vi "Untitled 2.vi"() -> ()   [LabVIEW 2018]
panel:
  in  "Action":enum16{"Create", "Fire", "Get", "Destroy"}(ring)=enum."Destroy"
  in  "Error In":errorcluster
  out "error out":errorcluster
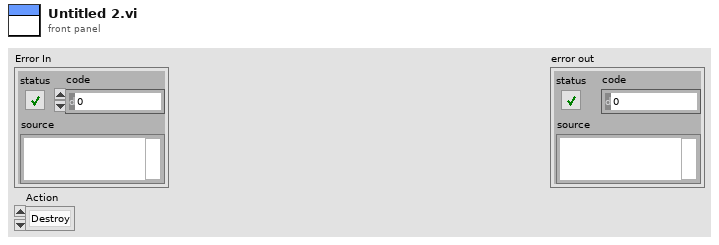
[diagram p1: front panel]
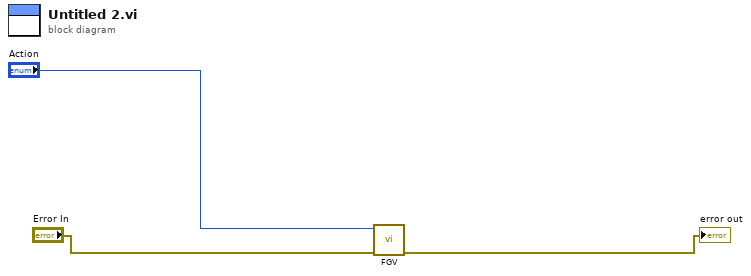
[diagram p0: block diagram]
diagram:
  n1 = call "FGV.vi"("error in"="Error In", 11:"Action") -> ("error out"=→"error out":errorcluster)  [unwired: 9 in]
